vi "sendCommand.vi"(8 "error in (no error)":errorcluster, 10 "Data in":u8[](array[numeric]), 11 "Command ID":u16 format="%04x") -> (0 "error out":errorcluster, 3 "Data out":u8[](array[numeric]))   [LabVIEW 2015, in "TPVG_DLL.lvlib"]
doc: "interacts with low level function to send command to and get reponse from AT-231 intrument.\n\n------------------------------------------\nAuthor: Dang Lam\nEmail: danglamtd@gmail.com"
uses:
  TPVG_DLL.lvlib
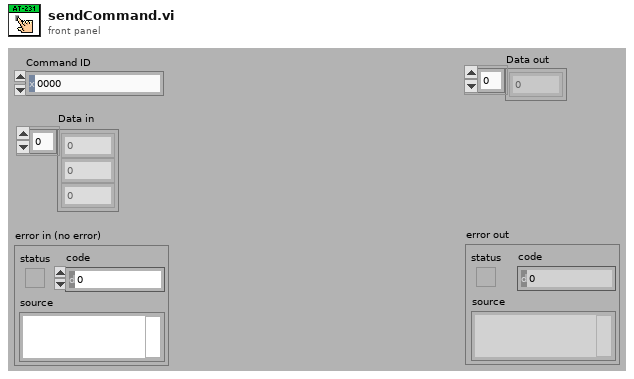
[diagram p1: front panel]
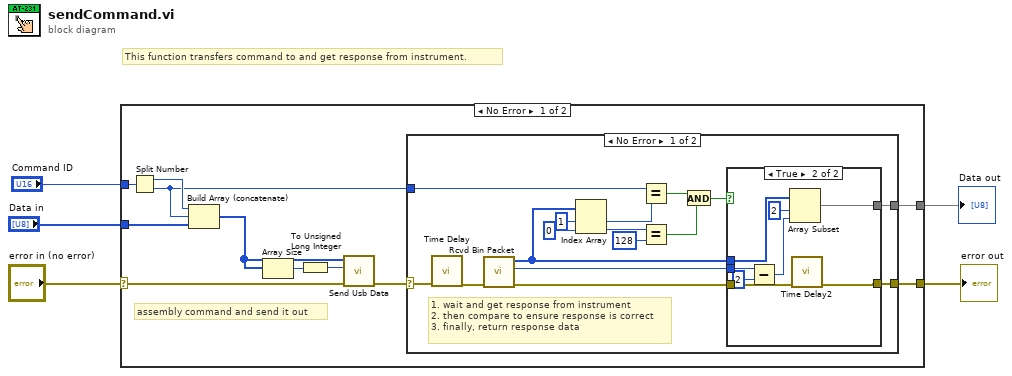
[diagram p0: block diagram]
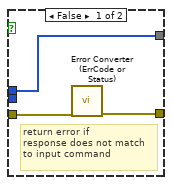
[diagram p2: hidden frame]
diagram:
  # "This function transfers command to and get response from instrument."
  n1 = case shown="No Error" "error in (no error)" {
    selector: "error in (no error)" -> [w15 w45]
    tunnel: [w7 w45] -> w4
    tunnel: "Command ID" -> [w16 _]
    tunnel: "Data in" -> [w14 _]
    tunnel: [w6 _] -> w1
    frame No Error {
      # "assembly command and send it out"
      n2 = Split Number(x=w16) -> (hi(x)=w9:u8, lo(x)=w8:u8)
      n3 = Build Array (concatenate)(w9, w8, w14) -> (w12:u8[])
      n4 = Array Size(array=w12) -> (size(s)=w13:i32)
      n5 = To Unsigned Long Integer(number=w13) -> (unsigned 32bit integer=w11:u32)
      n6 = call "Send Usb Data.vi"("error in (no error)"=w15, "Length"=w11, "Buffer"=w12) -> ("error out"=w10:errorcluster)  [unwired: 8 in]
      n7 = case shown="No Error" w10 {
        selector: w10 -> [w32 w44]
        tunnel: w8 -> [w28 _]
        tunnel: [w20 w44] -> w7
        tunnel: [w17 _] -> w6
        frame No Error {
          # "1. wait and get response from instrument \n2. then compare to ensure response is correct\n3. finally, return response data"
          n8 = call "Time Delay"("error in (no error)"=w32) -> ("error out"=w31:errorcluster)  [unwired: 10 in]
          n9 = call "Rcvd Bin Packet.vi"("error in (no error)"=w31) -> ("error out"=w21:errorcluster, "length"=w18:u32, "Buff"=w19:u8[])  [unwired: 8 in]
          n10 = Index Array(array=w19, index #1=1 ("index"), index #2=0 ("index")) -> (element #1=w27:u8, element #2=w26:u8)
          n11 = Equal?(x=w28, y=w27) -> (x = y?=w24:bool)
          n12 = Equal?(x=w26, y=u8 128) -> (x = y?=w23:bool)
          n13 = And(x=w24, y=w23) -> (x .and. y?=w22:bool)
          n14 = case shown="True" w22 {
            tunnel: w21 -> [w35 w36]
            tunnel: [w34 w37] -> w20
            tunnel: w19 -> [w33 w43]
            tunnel: w18 -> [_ w42]
            tunnel: [w33 w38] -> w17
            frame False {
              # "return error if\nresponse does not match\nto input command"
              n15 = call "Error Converter (ErrCode or Status).vi"("error in (no error)"=w35) -> ("error out"=w34:errorcluster)  [unwired: 10 in]
            }
            frame True {
              n16 = Subtract(x=w42, y=u32 2) -> (x-y=w40:u32)
              n17 = Array Subset(array=w43, index=2, length=w40) -> (w38:u8[])
              n18 = call "Time Delay2"("error in (no error)"=w36) -> ("error out"=w37:errorcluster)  [unwired: 10 in]
            }
          }
        }
        frame Error {
          # "skip and return error if any"
        }
      }
    }
    frame Error {
    }
  }
  "error out" <- w4
  "Data out" <- w1
